vi "DecayCluster2.vi"(0 "lifetime histograms":u32[][](array[numeric]), 1 "ch1 (0=sum)":i32, 2 "channel width (ns)":dbl format="%.2f", 3 "ch2":i32=1, 4 "ch3":i32=2) -> (5 "lifetime histograms":T1 {"channel width (ns)" format="%.2f"})   [LabVIEW 2009]
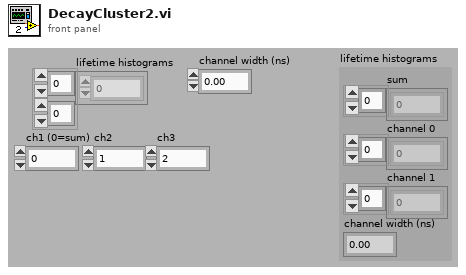
[diagram p1: front panel]
types:
  T1 = cluster{"sum":u32[], "channel 0":u32[], "channel 1":u32[], "channel width (ns)":dbl}
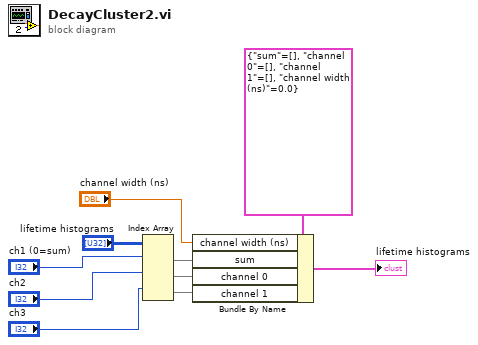
[diagram p0: block diagram]
diagram:
  n1 = Index Array(array="lifetime histograms", index (row) #1="ch1 (0=sum)", index (row) #2="ch2", index (row) #3="ch3") -> (element #1=w7:u32[], element #2=w8:u32[], element #3=w9:u32[])  [unwired: 3 in]
  n2 = Bundle By Name(cluster=T1 {"sum"=[], "channel 0"=[], "channel 1"=[], "channel width (ns)"=0.0}, "channel width (ns)"="channel width (ns)", "sum"=w7, "channel 0"=w8, "channel 1"=w9) -> (→"lifetime histograms":T1)
